vi "O-scope8.vi"() -> ()   [LabVIEW 2017]
uses:
  <vilib>/Waveform/WDTOps.llb/WDT Scale Delta t DBL.vi
  <vilib>/Waveform/WDTOps.llb/WDT Append Waveforms DBL.vi
panel:
  out "x-y":dbl
  out "voltage":dbl
  in  "rate":dbl=10000.0
  in  "number of samples":i32=10000
  in  "Tab Control":enum32{"Page 1", "Page 2", "Page 3"}(tab)
  out "Oscilloscope":waveform(dbl)(graph) caption="Waveform Graph"
  in  "volts/div":dbl(knob)=1.0 min=0.0 max=5.0 step=1.0 scale=5.0..1.0
  in  "Vert Pos":dbl(knob) min=-10.0 max=10.0 step=1.0 scale=-10.0..10.0
  in  "seconds/div":dbl(knob)=-1.0 min=-6.0 max=-1.0 step=1.0 scale=-6.0..-1.0 scale format="%#_9p"
  out "History":dynamicdata(graph)
  out "Waveform Graph":waveform(dbl)(graph)
  out "x*y 4":dbl
  out "x*y 3":dbl
  out "x*y 2":dbl
  out "x*y":dbl
  out "10^x":dbl
  in  "stop":bool=TRUE
  # "1m"
  # "100u"
  # "10m"
  # "10u"
  # "1u"
  # "100m"
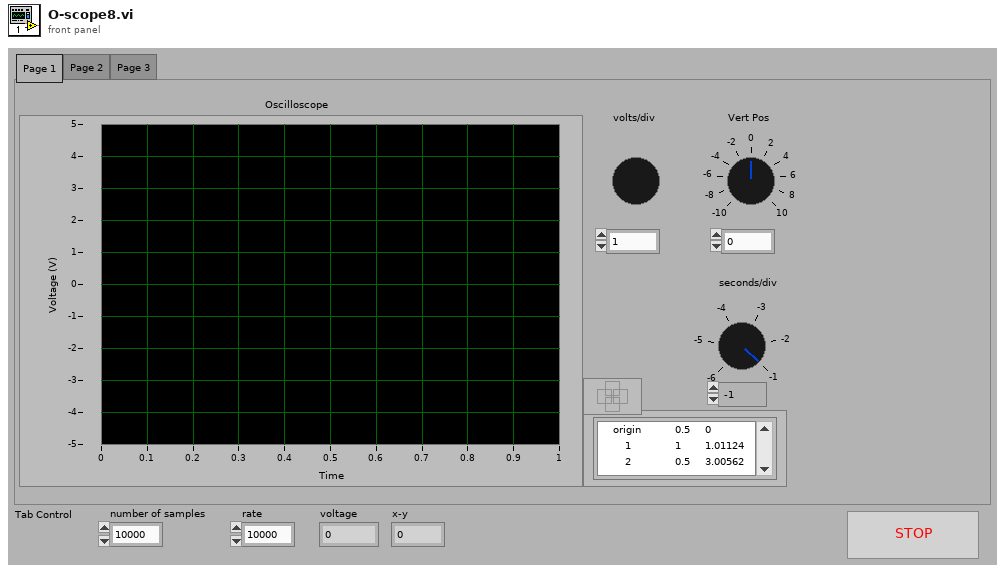
[diagram p1: front panel]
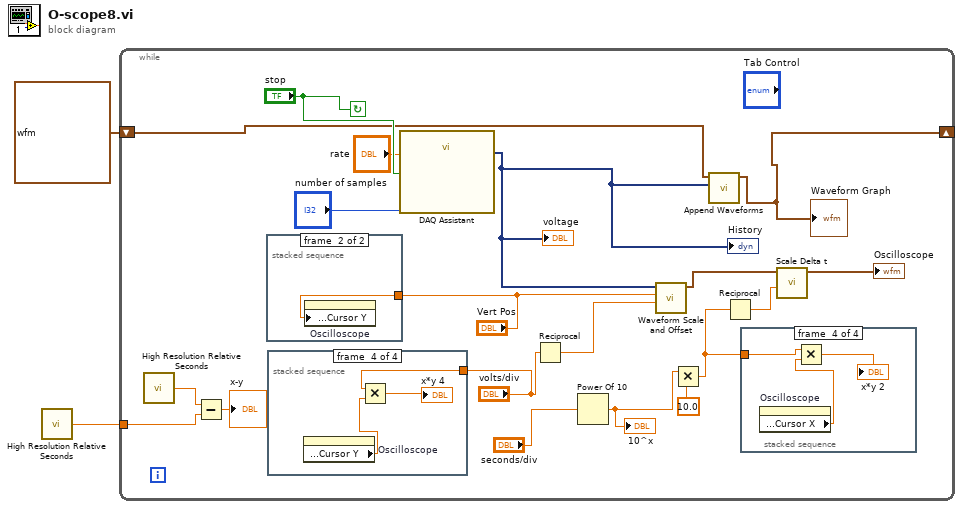
[diagram p0: block diagram]
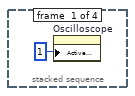
[diagram p2: hidden frame]
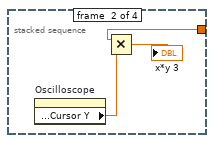
[diagram p3: hidden frame]
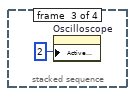
[diagram p4: hidden frame]
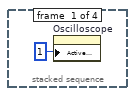
[diagram p5: hidden frame]
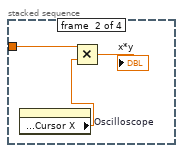
[diagram p6: hidden frame]
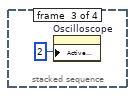
[diagram p7: hidden frame]
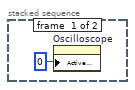
[diagram p8: hidden frame]
diagram:
  n1 = call <vilib>:"High Resolution Relative Seconds.vi"() -> ("relative seconds"=w1:dbl)
  n2 = while {
    shift-right: [w6] -> _
    shift-left: waveform(dbl) {"t0"=timestamp(0 s since 1904-01-01), "dt"=1.0, "Y"=[]} ("waveform out") -> [w8]
    tunnel: w1 -> [w4]
    stop <- "stop" continue-if-true
    n3 = call <vilib>:"High Resolution Relative Seconds.vi"() -> ("relative seconds"=w5:dbl)
    n4 = Subtract(x=w5, y=w4) -> (x-y=→"x-y":dbl)
    n5 = stacked-sequence {
      tunnel: "Vert Pos" -> [_ w39]
      frame #0 {
        n6 = property on="Oscilloscope" class="WFGraph (strict)"("Active Cursor"=u32 0) -> ()  [unwired: 2 in, 2 out]
      }
      frame #1 {
        n7 = property on="Oscilloscope" class="WFGraph (strict)"("Cursor.Cursor Position:Cursor Y"=w39) -> ()  [unwired: 2 in, 2 out]
      }
    }
    n8 = stacked-sequence {
      tunnel: "volts/div" -> [_ w24 _ w27]
      frame #0 {
        n9 = property on="Oscilloscope" class="WFGraph (strict)"("Active Cursor"=u32 1) -> ()  [unwired: 2 in, 2 out]
      }
      frame #1 {
        n10 = property on="Oscilloscope" class="WFGraph (strict)"() -> ("Cursor.Cursor Position:Cursor Y"=w23:dbl)  [unwired: 2 in, 2 out]
        n11 = Multiply(x=w24, y=w23) -> (x*y=→"x*y 3":dbl)
      }
      frame #2 {
        n12 = property on="Oscilloscope" class="WFGraph (strict)"("Active Cursor"=u32 2) -> ()  [unwired: 2 in, 2 out]
      }
      frame #3 {
        n13 = property on="Oscilloscope" class="WFGraph (strict)"() -> ("Cursor.Cursor Position:Cursor Y"=w28:dbl)  [unwired: 2 in, 2 out]
        n14 = Multiply(x=w27, y=w28) -> (x*y=→"x*y 4":dbl)
      }
    }
    n15 = call "DAQ Assistant"("rate"="rate", "number of samples"="number of samples", "stop (F)"="stop") -> ("data"=w7:dynamicdata)  [unwired: 13 in, 3 out]
    "voltage" <- w7
    "History" <- w7
    n16 = Reciprocal(x="volts/div") -> (1/x=w19:dbl)
    n17 = Power Of 10(x="seconds/div") -> (10^x=w17:dbl)
    "10^x" <- w17
    n18 = call <vilib>:"Waveform Scale and Offset.vi"("scale"=w19, "offset"="Vert Pos", "waveform in"=w7) -> ("waveform out"=w21:waveform(dbl))  [unwired: 7 in, 1 out]
    n19 = Multiply(x=w17, y=10.0) -> (x*y=w15:dbl)
    n20 = call-poly <vilib>:"Append Waveforms.vi"("waveform B"=w7, "waveform A"=w8) -> ("waveform out"=w6:waveform(dbl))  [unwired: 8 in, 1 out]
    "Waveform Graph" <- w6
    n21 = Reciprocal(x=w15) -> (1/x=w16:dbl)
    n22 = stacked-sequence {
      tunnel: w15 -> [_ w31 _ w35]
      frame #0 {
        n23 = property on="Oscilloscope" class="WFGraph (strict)"("Active Cursor"=u32 1) -> ()  [unwired: 2 in, 2 out]
      }
      frame #1 {
        n24 = property on="Oscilloscope" class="WFGraph (strict)"() -> ("Cursor.Cursor Position:Cursor X"=w33:dbl)  [unwired: 2 in, 2 out]
        n25 = Multiply(x=w31, y=w33) -> (x*y=→"x*y":dbl)
      }
      frame #2 {
        n26 = property on="Oscilloscope" class="WFGraph (strict)"("Active Cursor"=u32 2) -> ()  [unwired: 2 in, 2 out]
      }
      frame #3 {
        n27 = property on="Oscilloscope" class="WFGraph (strict)"() -> ("Cursor.Cursor Position:Cursor X"=w37:dbl)  [unwired: 2 in, 2 out]
        n28 = Multiply(x=w35, y=w37) -> (x*y=→"x*y 2":dbl)
      }
    }
    n29 = call-poly <vilib>:"Scale Delta t.vi"("scale factor"=w16, "waveform in"=w21) -> ("waveform out"=→"Oscilloscope":waveform(dbl))  [unwired: 8 in, 1 out]
  }
